vi "Method Descriptions.vi"(9 "OK Button":bool) -> ()   [LabVIEW 2022 SP3]
panel:
  in  "Method Descriptions":T1(tab)
  in  "String 19":string="Open Circuit Potential (OCP): Measures the electrochemical potential of the working electrode with respect to the reference electrode in the absence of an external load for the specified duration. The OCP is a measure of how far from equilibrium the species in solution are, and is determined by the Nernst equation. The OCP of solutions at equilibrium will vary little over time, while the OCP of solutions far from equilibrium will vary significantly with time."
  in  "String 21":string="Response"
  in  "String 18":string="Cyclic Voltammetry (CV): Measures the current response as the electrochemical potential of the working electrode is ramped linearly from Ei to the first vertex potential E1, is reversed to the second vertex potential E2, and back to Ei. The speed of the potential ramp is controlled by the scan rate, and the process can be repeated for a specified number of cycles. Cyclic voltammetry is the standard technique used to investigate the electrochemical properties of redox-active species in solution."
  in  "String 20":string="Experiment"
  in  "String 25":string="Response"
  in  "String 24":string="Experiment"
  in  "String 17":string="Linear Sweep Voltammetry (LSV): Measures the current response as the electrochemical potential of the working electrode is ramped linearly from Ei to Ef. The speed of the potential ramp is controlled by the scan rate. LSV is useful when studing electrochemical processes that are irreversible."
  in  "String 33":string="Response"
  in  "String 32":string="Experiment"
  in  "String 31":string="Anodic Stripping Voltammetry (ASV): ASV is useful for the quantitative determination of ionic species. The analyte of interest is first electroplated onto the working electrode during the deposition step, then oxidized from the electrode during the stripping step as the potential is ramped linearly from Ei to Ef. The current is measured during the stripping step, and is proportional to the concentration of the analyte in solution."
  in  "String 27":string="Response"
  in  "String 26":string="Experiment"
  in  "String 16":string="Chronoamperometry (CA): Measures the current response as a function of time after the working electrode potential is stepped to some applied potential Eap for the specified duration. The area under the i-t curve gives q, the total amount of charge passed to the working electrode, which in turn is related to the total number of electrons transferred by Faraday's constant. Chronoamperometry is useful for bulk electrolysis, whereby a given electrochemical reaction is driven by the applied potential."
  in  "String 30":string="Response"
  in  "String 29":string="Experiment"
  in  "String 28":string="Chronopotentiometry (CP): Measures the potential response as a function of time after the current at the working electrode is stepped to some applied current iap. Collection stops once the measured potential drops below the specified value or the experiment reaches the specified duration, whichever comes first. The total amount of charge produced is simply the product of the experiment duration and iap. Chronopotentiomatry is commonly used to evaluate the performance of batteries and fuel cells."
  in  "String 36":string="Response"
  in  "String 35":string="Experiment"
  in  "String 34":string="Galvanostatic Cycling: Measures the potential as a function of time as the cell is charged at some specified current then discharged at the same current. Collection stops once the experiment reaches the specified duration. This method is commonly used to evaluate the performance of rechargeable batteries and supercapacitors."
  in  "String 15":string="Ohmic Drop: The potential drop associated with the uncompensated solution resistance (the Ohmic drop, iRu) must be corrected for to ensure data free of distortions. This is done electronically through positive feedback circuitry.\n\nTo compensate for the Ohmic drop, observe the current response as the working electrode potential is repeatedly stepped to potential E2 while turning the compensation knob on the potentiostat. Once oscillations are observed, step back the knob. Disconnect the working electrode from the cell, click \"Measure Ru\", and adjust the knob to the specified amount of compensation, Rc."
  in  "String 22":string="Experiment"
  in  "String 23":string="Response"
  in  "String 14":string="Calibration: Records cyclic voltammetry for current response calibration of the potentiostat. Connect a resistor with a known resistance (the sample cell) between the working electrode and the reference/counter electrode. The i-V response gives a line with a slope that is equal to the known resistance according to Ohm's law. The slope is then used to calculate conversion factors the potentiostat uses to display electrochemical currents. To update the conversion factors, copy and paste the measured conversion factor into the conversion factor array."
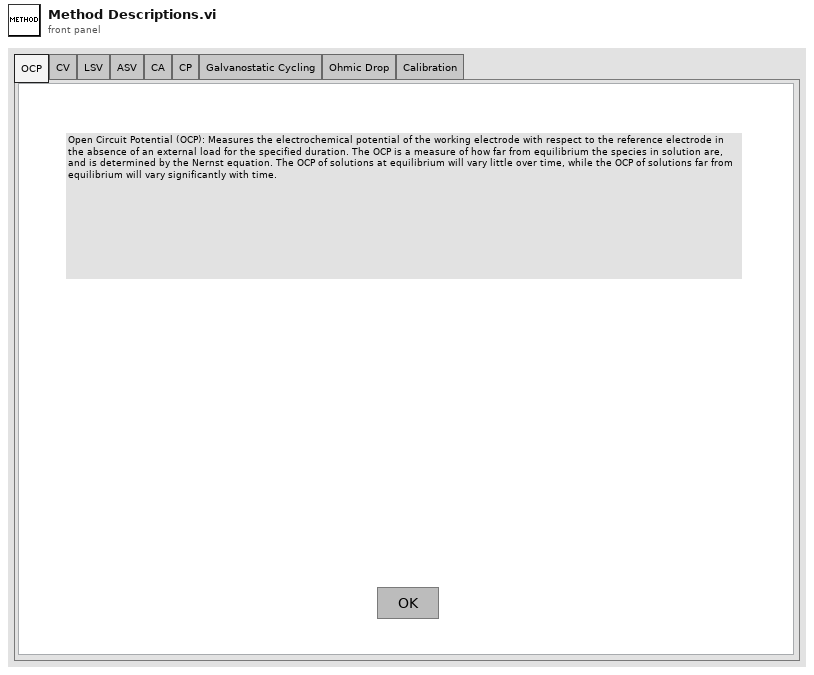
[diagram p1: front panel]
types:
  T1 = enum32{"OCP", "CV", "LSV", "ASV", "CA", "CP", "Galvanostatic Cycling", "Ohmic Drop", "Calibration"}
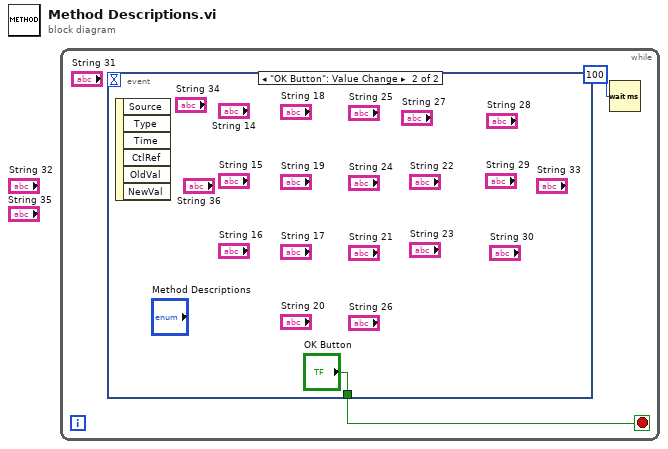
[diagram p0: block diagram]
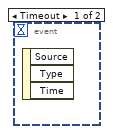
[diagram p2: hidden frame]
diagram:
  n1 = while {
    stop <- w2 stop-if-true
    n2 = event shown="[1] \"OK Button\": Value Change" {
      selector: _ -> [_ _]
      dyn-events: _ -> [_ _]
      timeout: _ -> [_ _]
      tunnel: [_ "OK Button"] -> w2
      event Timeout {
        n3 = event-data() -> ()  [unwired: 1 in, 3 out]
      }
      event "OK Button": Value Change {
        n4 = event-data() -> ()  [unwired: 1 in, 6 out]
      }
    }
    n5 = Wait (ms)(milliseconds to wait=u32 100) -> ()  [unwired: 1 out]
  }
